vi "checkRegCmdRule.vi"(8 "error in (no error)":errorcluster, 10 "packetConnID":T1, 11 "tcpServer in":refnum<class "TcpServer.lvclass">) -> (0 "error out":errorcluster, 1 "regCmd?":bool, 2 "packetConnID":T1, 3 "tcpServer out":refnum<class "TcpServer.lvclass">)   [LabVIEW 2018, in "TcpServer.lvclass"]
doc: "Check if command received is in the registered commands list. If is ok, it sends the commands as an user event to the User."
uses:
  TcpServer.lvclass
  typedef/packetConnIDTypeDef.ctl
  TcpServer.lvclass/TcpServer.ctl
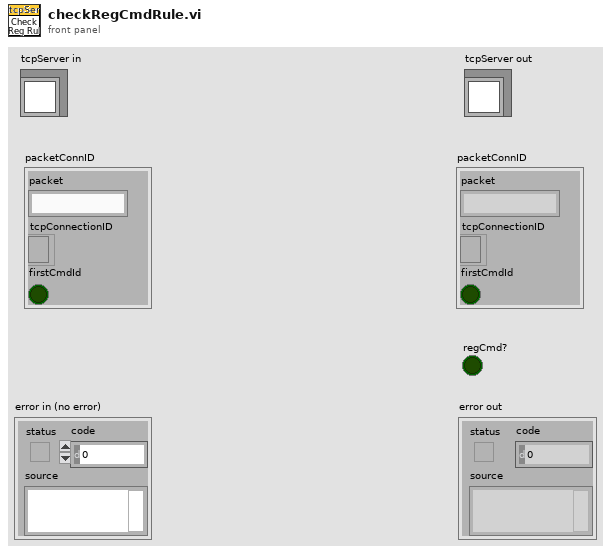
[diagram p1: front panel]
types:
  T1 = typedef "TcpServer.lvclass/packetConnIDTypeDef.ctl" = cluster{"packet":string, "tcpConnectionID":refnum<k5>, "firstCmdId":bool}
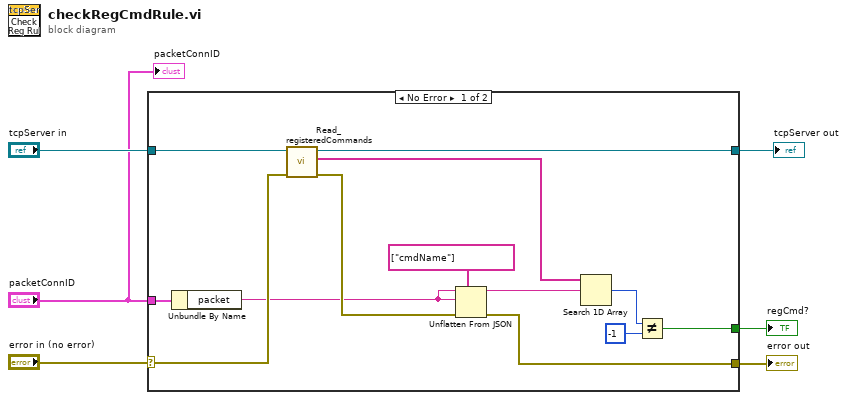
[diagram p0: block diagram]
diagram:
  n1 = case shown="No Error" "error in (no error)" {
    selector: "error in (no error)" -> [w10 w21]
    tunnel: [w14 w21] -> w3
    tunnel: [w11 w20] -> w4
    tunnel: "tcpServer in" -> [w13 w20]
    tunnel: [w17 _] -> w2
    tunnel: "packetConnID" -> [w8 _]
    frame No Error {
      n2 = Unbundle By Name(w8) -> ("packet"=w7:string)
      n3 = call "Read_registeredCommands.vi"("error in (no error)"=w10, "TcpServer in"=w13) -> ("error out"=w9:errorcluster, "registeredCommands"=w12:string[], "TcpServer out"=w11:refnum<class "TcpServer.lvclass">)  [unwired: 7 in]
      n4 = Unflatten From JSON(path=string[] ["cmdName"] ("tcp packet"), JSON string=w7, type and defaults=w7, error in (no error)=w9) -> (value=w15:string, error out=w14:errorcluster)  [unwired: 3 in]
      n5 = Search 1D Array(1D array=w12, element=w15) -> (index of element=w19:i32)  [unwired: 1 in]
      n6 = Not Equal?(x=w19, y=-1) -> (x != y?=w17:bool)
    }
    frame Error {
    }
  }
  "error out" <- w3
  "tcpServer out" <- w4
  "regCmd?" <- w2
  "packetConnID" <- "packetConnID"
